vi "Read Ex FPGA Ref.vi"(8 "error in (no error)":errorcluster, 11 "Exscalabar FPGA in":refnum<class "Exscalabar FPGA.lvclass">) -> (0 "error out":errorcluster, 2 "Ex FPGA Ref":T1, 3 "Exscalabar FPGA out":refnum<class "Exscalabar FPGA.lvclass">)   [LabVIEW 2014, in "Exscalabar FPGA.lvclass"]
uses:
  Exscalabar FPGA.lvclass
  R FPGA Ref.ctl
  Exscalabar FPGA.lvclass/Exscalabar FPGA.ctl
  PAS/ePAS Library.lvlib
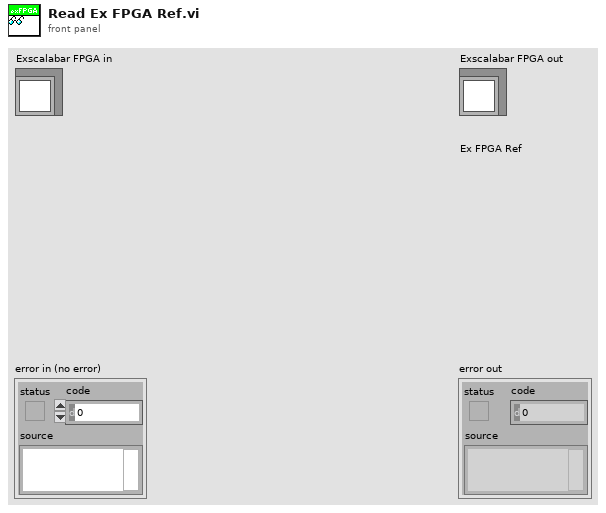
[diagram p1: front panel]
types:
  T1 = typedef "ePAS Library.lvlib/R FPGA Ref.ctl" = refnum<k20>
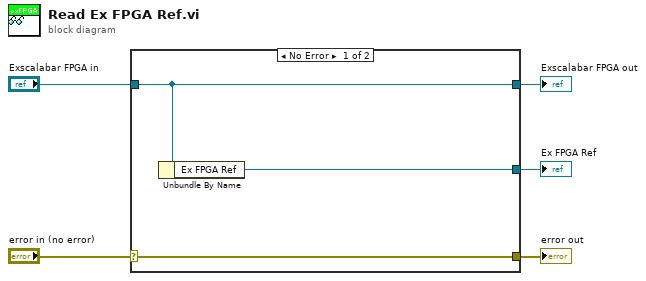
[diagram p0: block diagram]
diagram:
  n1 = case shown="No Error" "error in (no error)" {
    selector: "error in (no error)" -> [w8 w9]
    tunnel: [w8 w9] -> w4
    tunnel: [w7 w10] -> w2
    tunnel: "Exscalabar FPGA in" -> [w7 w10]
    tunnel: [w6 _] -> w1
    frame No Error {
      n2 = Unbundle By Name(w7) -> ("Ex FPGA Ref"=w6:T1)
    }
    frame Error {
    }
  }
  "error out" <- w4
  "Exscalabar FPGA out" <- w2
  "Ex FPGA Ref" <- w1
